vi "SW_Gen_Draw_Segments_DAQmx.vi"(6 "Colors cluster":T3, 7 "Show magnets":bool, 8 "Cluster of image geometrical and scaling parameters":T1, 9 "Input cluster of parameters":T4={"Amount of border segments"=8, "Border segments starting angle"=0, "Amount of midfield segments"=4, "Midfield segments starting angle"=0, "Midfield segments outer radius, mm"=60, "Amount of central segments"=1, "Center segment outer radius, mm"=30, "Diameter of the cage, mm"=180, "R-gap between segments, mm"=10} {"Diameter of the cage, mm" scale=20.0..250.0}, 10 "Bounding rectangles":T2, 11 "Zones display background in":picture) -> (1 "Array of the pixel to color correspondences":u32[][](array[numeric]), 2 "No zones image":picture, 3 "Zones in the cage layout":picture)   [LabVIEW 2018]
panel:
  in  "Color of the South magnet":u32(colorbox)=9567230
  in  "Color of the North magnet":u32(colorbox)=16711680
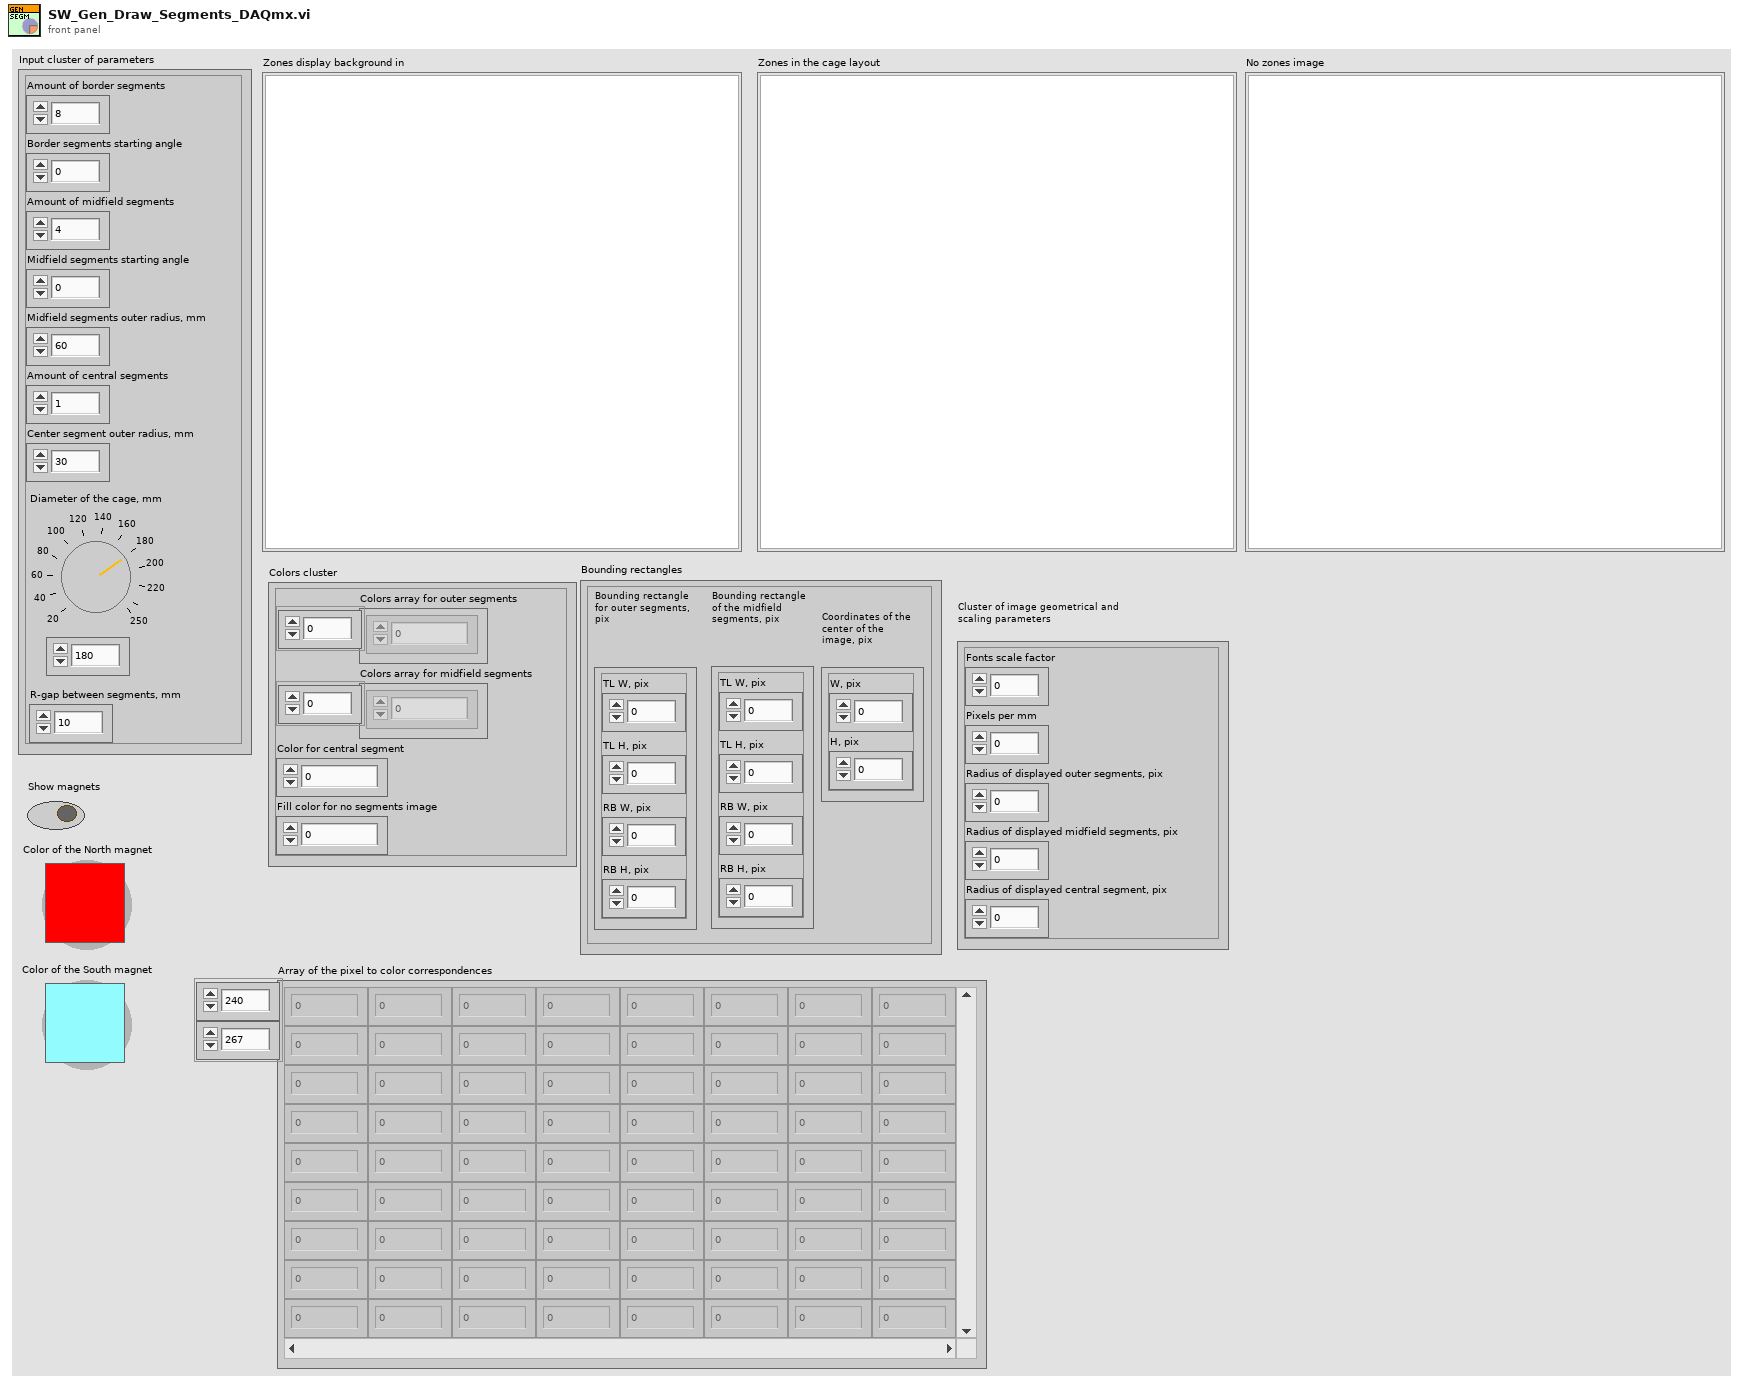
[diagram p1: front panel]
types:
  T1 = cluster{"Fonts scale factor":dbl, "Pixels per mm":dbl, "Radius of displayed outer segments, pix":dbl, "Radius of displayed midfield segments, pix":dbl, "Radius of displayed central segment, pix":dbl}
  T2 = cluster{"Bounding rectangle for outer segments, pix":cluster{"TL W, pix":dbl, "TL H, pix":dbl, "RB W, pix":dbl, "RB H, pix":dbl}, "Bounding rectangle of the midfield segments, pix":cluster{"TL W, pix":dbl, "TL H, pix":dbl, "RB W, pix":dbl, "RB H, pix":dbl}, "Coordinates of the center of the image, pix":cluster{"W, pix":dbl, "H, pix":dbl}}
  T3 = cluster{"Colors array for outer segments":u32[], "Colors array for midfield segments":u32[], "Color for central segment":u32, "Fill color for no segments image":u32}
  T4 = cluster{"Amount of border segments":u8, "Border segments starting angle":i16, "Amount of midfield segments":u8, "Midfield segments starting angle":i16, "Midfield segments outer radius, mm":u16, "Amount of central segments":u8, "Center segment outer radius, mm":u16, "Diameter of the cage, mm":u16, "R-gap between segments, mm":u8}
  T5 = cluster{"Width":u16, "Style":enum32{"Solid", "Dash", "Dot", "DashDot", "DashDotDot"}}
  T6 = cluster{"TL W, pix":dbl, "TL H, pix":dbl, "RB W, pix":dbl, "RB H, pix":dbl}
  T7 = typedef "imagedata.ctl" = cluster{"image type":i32, "image depth":i32, "image":u8[], "mask":u8[], "colors":u32[], "Rectangle":cluster{"left":i16, "top":i16, "right":i16, "bottom":i16}}
  T8 = cluster{"left":i16, "top":i16, "right":i16, "bottom":i16}
  T9 = cluster{"image[0]":u8, "image[1]":u8, "image[2]":u8}
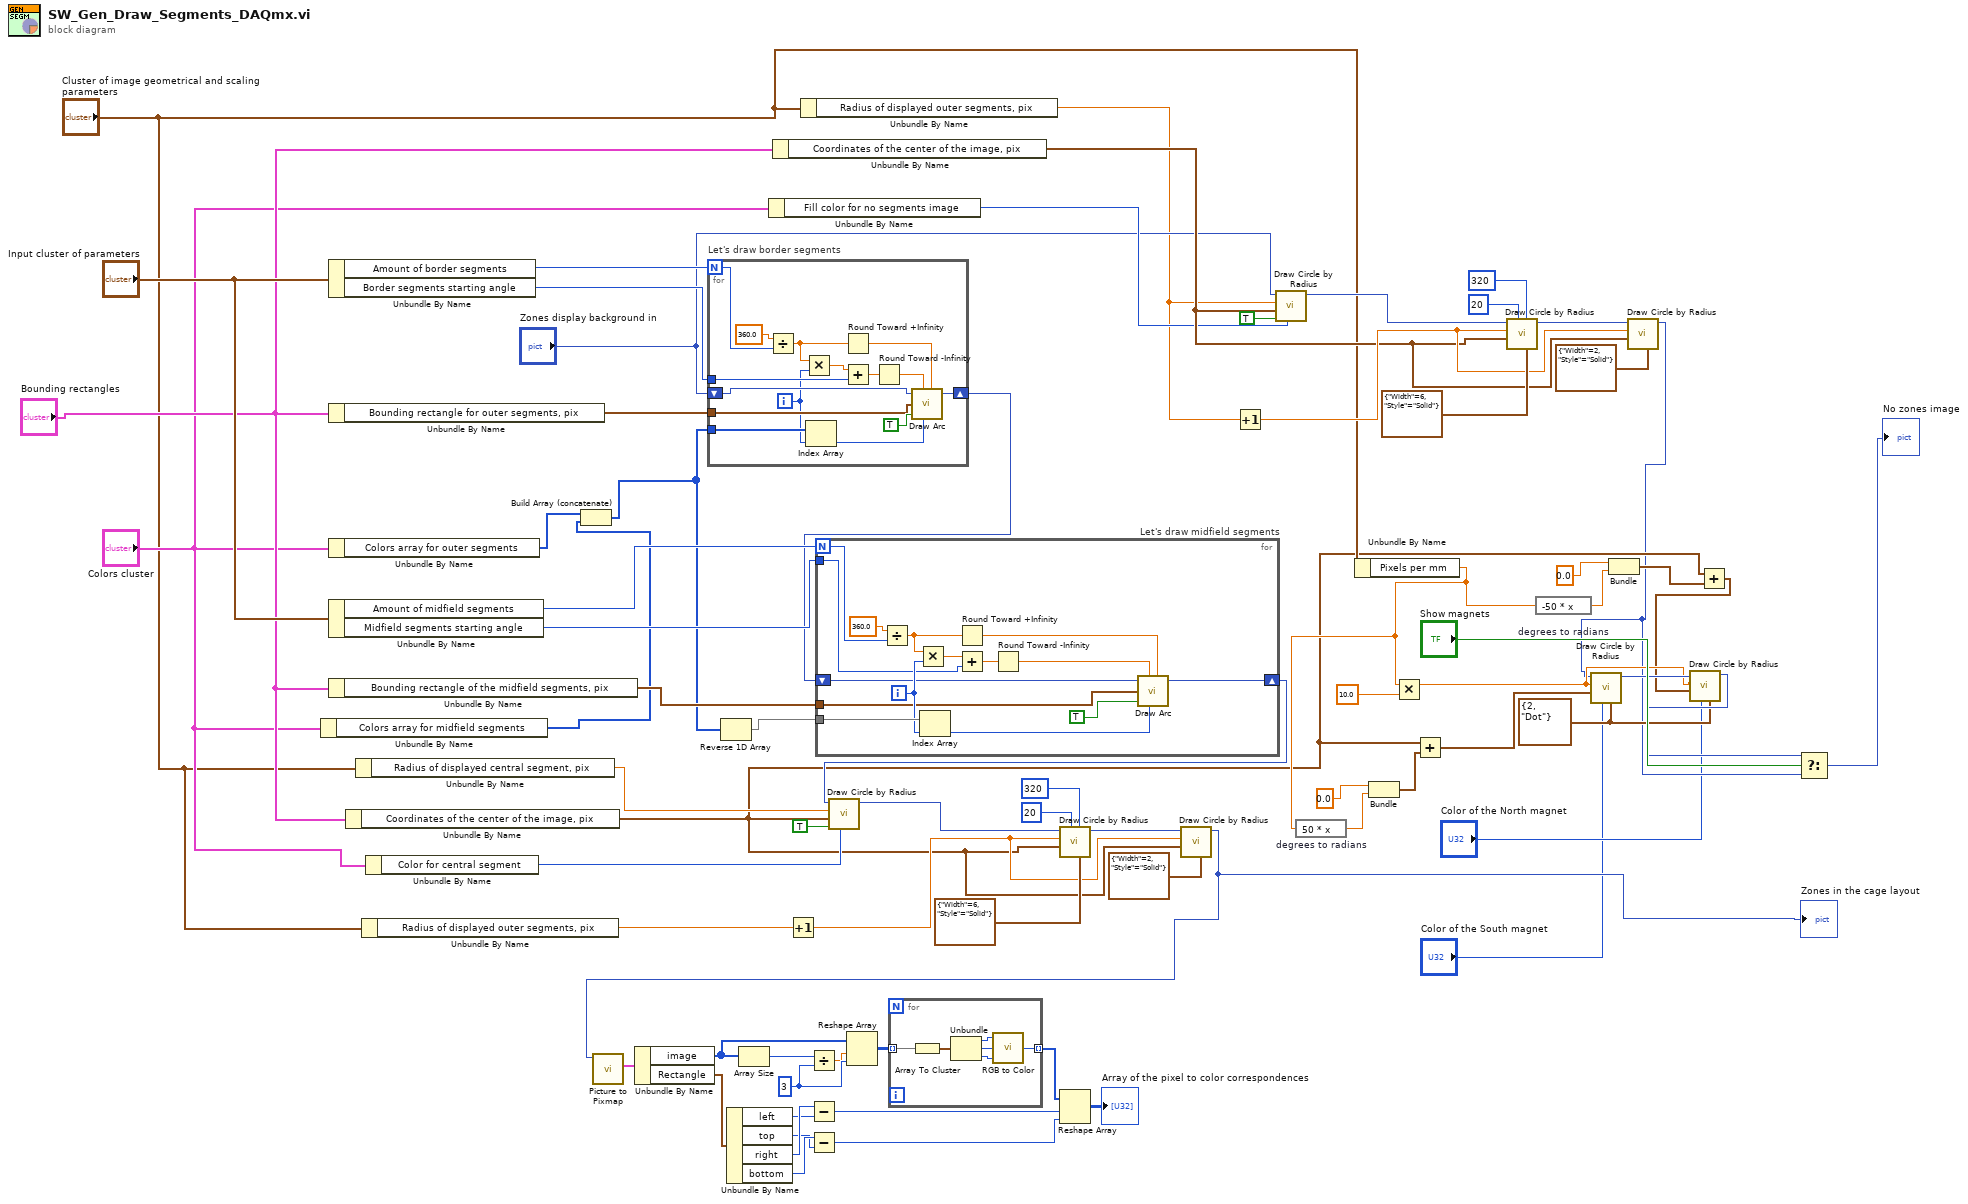
[diagram p0: block diagram]
diagram:
  w18 = T5 {"Width"=2, "Style"=enum."Dot"} ("pen")
  w53 = 3 ("dimension size")
  n1 = Unbundle By Name("Colors cluster") -> ("Colors array for midfield segments"=w4:u32[])
  n2 = Unbundle By Name("Input cluster of parameters") -> ("Amount of border segments"=w75:u8, "Border segments starting angle"=w74:i16)
  n3 = Unbundle By Name("Bounding rectangles") -> ("Bounding rectangle for outer segments, pix"=w73:T6)
  n4 = Unbundle By Name("Colors cluster") -> ("Colors array for outer segments"=w3:u32[])
  n5 = Unbundle By Name("Input cluster of parameters") -> ("Amount of midfield segments"=w72:u8, "Midfield segments starting angle"=w71:i16)
  n6 = Unbundle By Name("Bounding rectangles") -> ("Bounding rectangle of the midfield segments, pix"=w69:T6)
  n7 = Unbundle By Name("Bounding rectangles") -> ("Coordinates of the center of the image, pix"=w12:cluster{"W, pix":dbl, "H, pix":dbl})
  n8 = Unbundle By Name("Cluster of image geometrical and scaling parameters") -> ("Radius of displayed central segment, pix"=w28:dbl)
  n9 = Unbundle By Name("Cluster of image geometrical and scaling parameters") -> ("Radius of displayed outer segments, pix"=w58:dbl)
  n10 = Unbundle By Name("Colors cluster") -> ("Color for central segment"=w67:u32)
  n11 = Build Array (concatenate)(w3, w4) -> (w2:u32[])
  n12 = for "Let's draw border segments" {
    N: w75 -> [w82]
    tunnel: w74 -> [w87]
    shift-right: [w80] -> w70
    shift-left: "Zones display background in" -> [w89]
    tunnel: w73 -> [w83]
    tunnel: w2 -> [w86]
    i -> [w77]
    n13 = Divide(x=360.0, y=w82) -> (x/y=w81:dbl)
    n14 = Multiply(x=w81, y=w77) -> (x*y=w88:dbl)
    n15 = Index Array(array=w86, index=w77) -> (element=w76:u32)
    n16 = Round Toward +Infinity(x=w81) -> (ceil(x): smallest int >= x=w79:dbl)
    n17 = Add(x=w88, y=w87) -> (x+y=w84:dbl)
    n18 = Round Toward -Infinity(1:w84) -> (0:w78:dbl)
    n19 = call <vilib>:"Draw Arc.vi"("picture"=w89, "start angle[degrees]"=w78, "rect"=w83, "fill?(F)"=TRUE, "color(black)"=w76, "arc size[degrees]"=w79) -> ("new picture"=w80:picture)  [unwired: 3 in]
  }
  n20 = Reverse 1D Array(array=w2) -> (reversed array=w1:u32[])
  n21 = Unbundle By Name("Colors cluster") -> ("Fill color for no segments image"=w30:u32)
  n22 = Unbundle By Name("Bounding rectangles") -> ("Coordinates of the center of the image, pix"=w32:cluster{"W, pix":dbl, "H, pix":dbl})
  n23 = Increment(x=w58) -> (x+1=w57:dbl)
  n24 = Unbundle By Name("Cluster of image geometrical and scaling parameters") -> ("Radius of displayed outer segments, pix"=w25:dbl)
  n25 = for "Let's draw midfield segments" {
    N: w72 -> [w96]
    shift-right: [w91] -> w68
    shift-left: w70 -> [w92]
    tunnel: w71 -> [w94]
    tunnel: w69 -> [w93]
    tunnel: w1 -> [w98]
    i -> [w95]
    n26 = Divide(x=360.0, y=w96) -> (x/y=w100:dbl)
    n27 = Multiply(x=w100, y=w95) -> (x*y=w101:dbl)
    n28 = Index Array(array=w98, index=w95) -> (element=w97:u32)
    n29 = Round Toward +Infinity(x=w100) -> (ceil(x): smallest int >= x=w103:dbl)
    n30 = Add(x=w101, y=w94) -> (x+y=w102:dbl)
    n31 = Round Toward -Infinity(1:w102) -> (0:w104:dbl)
    n32 = call <vilib>:"Draw Arc.vi"("picture"=w92, "start angle[degrees]"=w104, "rect"=w93, "fill?(F)"=TRUE, "color(black)"=w97, "arc size[degrees]"=w103) -> ("new picture"=w91:picture)  [unwired: 3 in]
  }
  n33 = call <vilib>:"Draw Circle by Radius.vi"("color(black)"=w67, "fill?(F)"=TRUE, "pixel center"=w12, "radius"=w28, "picture"=w68) -> ("new picture"=w59:picture)  [unwired: 6 in]
  n34 = call <vilib>:"Draw Circle by Radius.vi"("pen"=T5 {"Width"=6, "Style"=enum."Solid"}, "arc size(360)"=i16 320, "start angle(0)"=i16 20, "pixel center"=w12, "radius"=w57, "picture"=w59) -> ("new picture"=w64:picture)  [unwired: 5 in]
  n35 = call <vilib>:"Draw Circle by Radius.vi"("pen"=T5 {"Width"=2, "Style"=enum."Solid"}, "pixel center"=w12, "radius"=w57, "picture"=w64) -> ("new picture"=w9:picture)  [unwired: 7 in]
  "Zones in the cage layout" <- w9
  n36 = call <vilib>:"Picture to Pixmap.vi"("picture"=w9) -> ("image data"=w56:T7)  [unwired: 9 in, 1 out]
  n37 = Unbundle By Name(w56) -> ("image"=w55:u8[], "Rectangle"=w50:T8)
  n38 = Unbundle By Name(w50) -> ("left"=w47:i16, "top"=w44:i16, "right"=w48:i16, "bottom"=w45:i16)
  n39 = Array Size(array=w55) -> (size(s)=w54:i32)
  n40 = Divide(x=w54, y=w53) -> (x/y=w52:dbl)
  n41 = Subtract(x=w48, y=w47) -> (x-y=w46:i16)
  n42 = Subtract(x=w45, y=w44) -> (x-y=w43:i16)
  n43 = Reshape Array(w55, w52, w53) -> (w51:u8[][])
  n44 = for {
    tunnel: w51 -> [w111] mode=indexing
    tunnel: [w106] -> w49 mode=indexing
    n45 = Array To Cluster(array=w111) -> (cluster=w110:T9)
    n46 = Unbundle(w110) -> ("image[0]"=w109:u8, "image[1]"=w108:u8, "image[2]"=w107:u8)
    n47 = call <vilib>:"RGB to Color.vi"("B"=w107, "G"=w108, "R"=w109) -> ("Color"=w106:u32)
  }
  n48 = Reshape Array(w49, w46, w43) -> (→"Array of the pixel to color correspondences":u32[][])
  n49 = Increment(x=w25) -> (x+1=w34:dbl)
  n50 = call <vilib>:"Draw Circle by Radius.vi"("color(black)"=w30, "fill?(F)"=TRUE, "pixel center"=w32, "radius"=w25, "picture"="Zones display background in") -> ("new picture"=w35:picture)  [unwired: 6 in]
  n51 = Unbundle By Name("Cluster of image geometrical and scaling parameters") -> ("Pixels per mm"=w13:dbl)
  n52 = expression code="50 * x" "degrees to radians"(w13) -> (w22:dbl)
  n53 = Bundle("W, pix"=0.0, "Pixels per mm"=w22) -> (w21:cluster{"W, pix":dbl, "Pixels per mm":dbl})  [unwired: 1 in]
  n54 = Multiply(x=w13, y=10.0) -> (x*y=w17:dbl)
  n55 = Add(x=w12, y=w21) -> (x+y=w16:cluster{"W, pix":dbl, dbl})
  n56 = call <vilib>:"Draw Circle by Radius.vi"("pen"=T5 {"Width"=6, "Style"=enum."Solid"}, "arc size(360)"=i16 320, "start angle(0)"=i16 20, "pixel center"=w32, "radius"=w34, "picture"=w35) -> ("new picture"=w40:picture)  [unwired: 5 in]
  n57 = expression code="-50 * x" "degrees to radians"(w13) -> (w14:dbl)
  n58 = Bundle("W, pix"=0.0, "Pixels per mm"=w14) -> (w11:cluster{"W, pix":dbl, "Pixels per mm":dbl})  [unwired: 1 in]
  n59 = call <vilib>:"Draw Circle by Radius.vi"("pen"=T5 {"Width"=2, "Style"=enum."Solid"}, "pixel center"=w32, "radius"=w34, "picture"=w40) -> ("new picture"=w7:picture)  [unwired: 7 in]
  n60 = call <vilib>:"Draw Circle by Radius.vi"("pen"=w18, "color(black)"="Color of the South magnet", "pixel center"=w16, "radius"=w17, "picture"=w7) -> ("new picture"=w20:picture)  [unwired: 6 in]
  n61 = Add(x=w12, y=w11) -> (x+y=w10:cluster{"W, pix":dbl, dbl})
  n62 = call <vilib>:"Draw Circle by Radius.vi"("pen"=w18, "color(black)"="Color of the North magnet", "pixel center"=w10, "radius"=w17, "picture"=w20) -> ("new picture"=w19:picture)  [unwired: 6 in]
  n63 = Select(t=w19, s="Show magnets", f=w7) -> (s? t:f=→"No zones image":picture)
